vi "Open or Create Polymorphic VI.vi"(6 "Description":string, 8 "error in (no error)":errorcluster, 9 "Owner":refnum<vi>, 10 "Icon":refnum<class "Icon.lvclass">, 11 "Polymorphic VI Path In":path) -> (0 "error out":errorcluster, 2 "Polymorphic Library Owner":refnum<vi>, 3 "Polymorphic VI Refnum":refnum<vi>)   [LabVIEW 2020]
doc: "Opens or creates a new polymorphic VI, setting the icon, description, and library owner."
uses:
  <vilib>/LabVIEW Icon API/lv_icon/Classes/Icon/Icon.lvclass
  <vilib>/LabVIEW Icon API/LabVIEW Icon API.lvlib
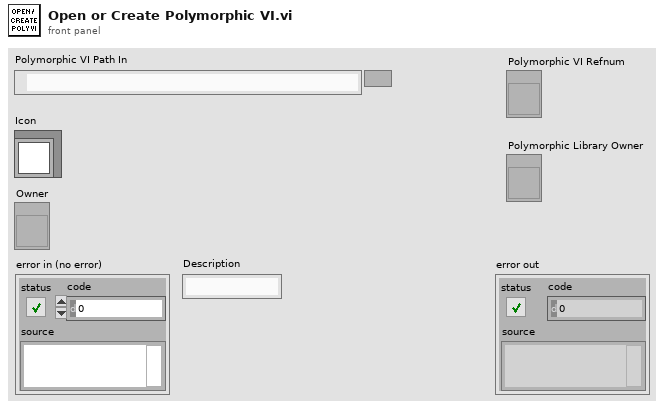
[diagram p1: front panel]
types:
  T1 = enum32{"invalid VI type", "Standard VI", "Control VI", "Global VI", "Polymorphic VI", "Configuration VI", "SubSystem", "Facade VI", "Method VI", "Statechart Diagram VI"}
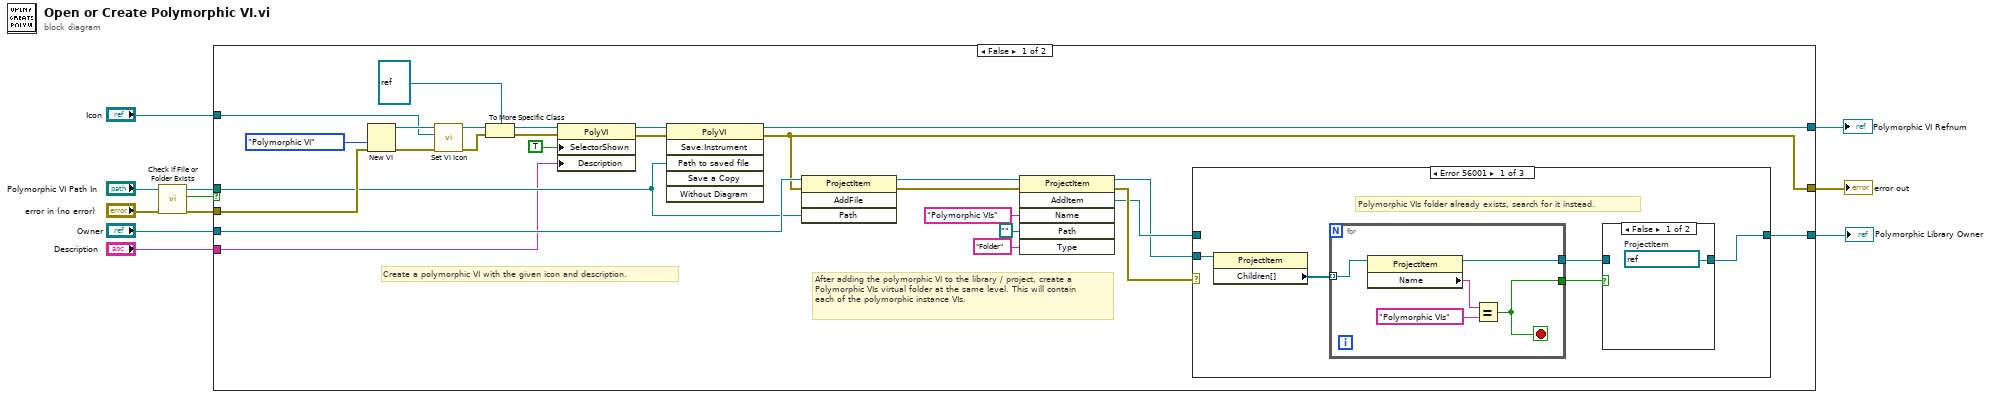
[diagram p0: block diagram]
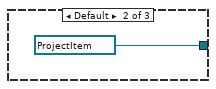
[diagram p3: hidden frame]
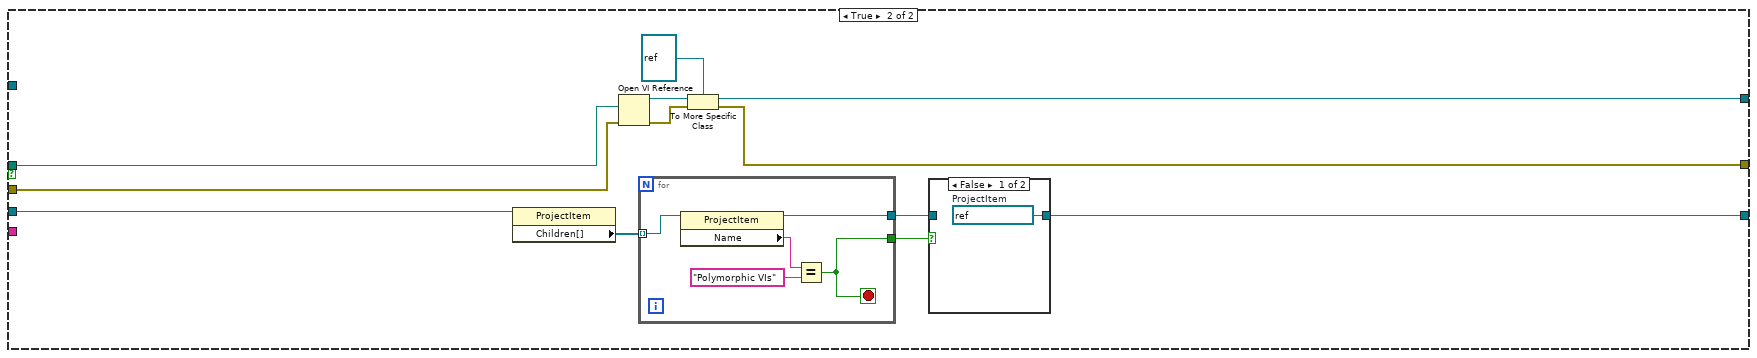
[diagram p5: hidden frame]
diagram:
  n1 = call <vilib>:"Check if File or Folder Exists.vi"("error in (no error)"="error in (no error)", "path"="Polymorphic VI Path In") -> ("error out"=w6:errorcluster, "file or folder exists?"=w10:bool, "dup path"=w9:path)  [unwired: 7 in]
  n2 = case shown="False" w10 {
    tunnel: w9 -> [w23 w64]
    tunnel: [w31 w58] -> w8
    tunnel: w6 -> [w30 w61]
    tunnel: [w13 w59] -> w5
    tunnel: "Icon" -> [w25 _]
    tunnel: "Owner" -> [w24 w57]
    tunnel: "Description" -> [w22 _]
    tunnel: [w16 w54] -> w1
    frame False {
      # "After adding the polymorphic VI to the library / project, create a Polymorphic VIs virtual folder at the same level. This will contain each of the polymorphic instance VIs."
      # "Create a polymorphic VI with the given icon and description."
      n3 = New VI(8:w30, 9:T1."Polymorphic VI" ("vi type (standard vi)")) -> (0:w28:errorcluster, 3:w29:refnum<vi>)  [unwired: 5 in]
      n4 = call <vilib>:"Set VI Icon.vi"("error in (no error)"=w28, "Icon"=w25, "VI Refnum in"=w29) -> ("error out"=w27:errorcluster, "VI Refnum out"=w26:refnum<vi>)  [unwired: 7 in]
      n5 = To More Specific Class(target class=refnum<vi> refnum ("vi refnum"), reference=w26, error in=w27) -> (specific class reference=w36:refnum<vi>, error out=w33:errorcluster)
      n6 = property on="Property Node" class="PolyVI"(reference=w36, error in=w33, "SelectorShown"=TRUE ("Show Selector By Default"), "Description"=w22) -> (reference out=w35:refnum<vi>, error out=w32:errorcluster)
      n7 = invoke on="Invoke Node" class="PolyVI" method="Save.Instrument"(reference=w35, error in=w32, "Path to saved file"=w23) -> (reference out=w31:refnum<vi>, error out=w13:errorcluster)  [unwired: 3 in, 4 out]
      n8 = invoke on="Invoke Node" class="ProjectItem" method="AddFile"(reference=w24, error in=w13, "Path"=w23) -> (reference out=w21:refnum<vi>, error out=w20:errorcluster)  [unwired: 1 in, 2 out]
      n9 = invoke on="Invoke Node" class="ProjectItem" method="AddItem"(reference=w21, error in=w20, "Name"="Polymorphic VIs", "Path"=path "" ("Empty Path Constant"), "Type"="Folder") -> (reference out=w12:refnum<vi>, error out=w15:errorcluster, "AddItem"=w14:refnum<vi>)  [unwired: 1 in, 3 out]
      n10 = case shown="Error 56001" w15 {
        tunnel: [w40 refnum<vi> refnum ("AddItem") w52] -> w16
        tunnel: w14 -> [_ _ w52]
        tunnel: w12 -> [w39 _ _]
        frame Error {
          # "Polymorphic VIs folder already exists, search for it instead."
          n11 = property on="Property Node" class="ProjectItem"(reference=w39) -> ("Children[]"=w43:refnum<vi>[])  [unwired: 1 in, 2 out]
          n12 = for {
            tunnel: w43 -> [w50] mode=indexing
            tunnel: [w47] -> w41
            tunnel: [w46] -> w42
            stop <- w46 stop-if-true
            n13 = property on="Property Node" class="ProjectItem"(reference=w50) -> (reference out=w47:refnum<vi>, "Name"=w49:string)  [unwired: 1 in, 1 out]
            n14 = Equal?(x=w49, y="Polymorphic VIs") -> (x = y?=w46:bool)
          }
          n15 = case shown="False" w42 {
            tunnel: [w44 w45] -> w40
            tunnel: w41 -> [_ w45]
            frame False {
              w44 = refnum<vi> refnum  # ProjectItem
            }
            frame True {
            }
          }
        }
        frame Default {
        }
        frame No Error {
        }
      }
    }
    frame True {
      n16 = property on="Property Node" class="ProjectItem"(reference=w57) -> ("Children[]"=w56:refnum<vi>[])  [unwired: 1 in, 2 out]
      n17 = Open VI Reference(vi path=w64, error in (no error)=w61) -> (vi reference=w62:refnum<vi>, error out=w60:errorcluster)  [unwired: 4 in]
      n18 = for {
        tunnel: w56 -> [w71] mode=indexing
        tunnel: [w68] -> w53
        tunnel: [w67] -> w55
        stop <- w67 stop-if-true
        n19 = property on="Property Node" class="ProjectItem"(reference=w71) -> (reference out=w68:refnum<vi>, "Name"=w70:string)  [unwired: 1 in, 1 out]
        n20 = Equal?(x=w70, y="Polymorphic VIs") -> (x = y?=w67:bool)
      }
      n21 = To More Specific Class(target class=refnum<vi> refnum ("vi refnum"), reference=w62, error in=w60) -> (specific class reference=w58:refnum<vi>, error out=w59:errorcluster)
      n22 = case shown="False" w55 {
        tunnel: [w65 w66] -> w54
        tunnel: w53 -> [_ w66]
        frame False {
          w65 = refnum<vi> refnum  # ProjectItem
        }
        frame True {
        }
      }
    }
  }
  "Polymorphic VI Refnum" <- w8
  "error out" <- w5
  "Polymorphic Library Owner" <- w1
